vi "Threshold.vi"(3 "Error":string, 4 "Threshold":i16, 5 "Output Image":T1={"Image ID"=0, "Channel ID"=-1}, 6 "Input Image":T1={"Image ID"=0, "Channel ID"=-1}) -> (0 "Error":string, 1 "Output Image":T1={"Image ID"=0, "Channel ID"=-1}, 2 "Input Image":T1={"Image ID"=0, "Channel ID"=-1})   [LabVIEW 2011, in "labvvis.lvlib"]
doc: "Each pixel in Input Image is compared with Threshold. If the pixel is greater than the Threshold, then the result is 255 (0xFF). Otherwise, the result is 0. The result is written to the Output Image."
uses:
  <userlib>/labvvis/labvvis.lvlib
  <userlib>/labvvis/VVIS Image.ctl
  labvvis.framework
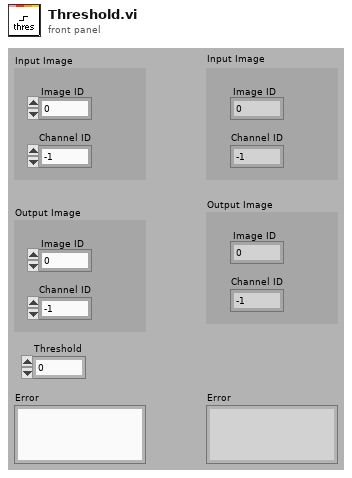
[diagram p1: front panel]
types:
  T1 = typedef "labvvis.lvlib/VVIS Image.ctl" = cluster{"Image ID":i16, "Channel ID":i16}
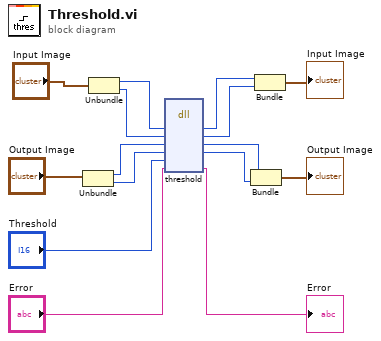
[diagram p0: block diagram]
diagram:
  n1 = Unbundle("Output Image") -> ("Image ID"=w11:i16, "Channel ID"=w10:i16)
  n2 = Unbundle("Input Image") -> ("Image ID"=w14:i16, "Channel ID"=w12:i16)
  n3 = dll-call lib="labvvis.framework" fn="threshold"("src1"=w14, "cid"=w12, "out"=w11, "ocid"=w10, "value"="Threshold", "Error") -> ("src1"=w3:i16, "cid"=w4:i16, "out"=w5:i16, "ocid"=w6:i16, →"Error":string)  [unwired: 5 in, 2 out]
  n4 = Bundle("out"=w5, "ocid"=w6) -> (→"Output Image":cluster{"out":i16, "ocid":i16})  [unwired: 1 in]
  n5 = Bundle("src1"=w3, "cid"=w4) -> (→"Input Image":cluster{"src1":i16, "cid":i16})  [unwired: 1 in]
